vi "Is Over-Range.vi"(8 "error in (no error)":errorcluster, 10 "measurement value":dbl format="%^.2e", 11 "CS++DMM in":refnum<class "CS++DMM.lvclass">) -> (0 "error out":errorcluster, 2 "is over-range":bool, 3 "CS++DMM out":refnum<class "CS++DMM.lvclass">)   [LabVIEW 2015, in "CS++DMM.lvlib" / "CS++DMM.lvclass"]
doc: "This VI takes a measurement value that you obtain from either the Read or Fetch VIs and determines if the value is a valid measurement value or a value indicating that an over-range condition occurred. \n\nNotes:\n\n(1) If an over-range condition occurs, the measurement value contains an IEEE defined NaN (Not a Number) value indicating that an over-range condition occurred.\n\n(2) This VI does not check the instrument status."
uses:
  CS++DMM.lvclass
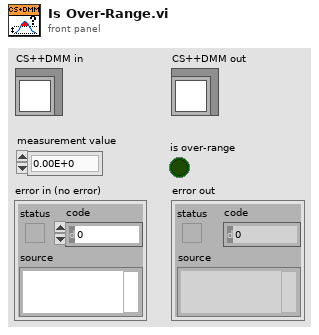
[diagram p1: front panel]
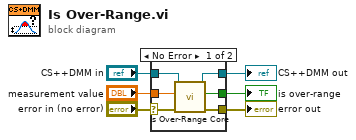
[diagram p0: block diagram]
diagram:
  n1 = case shown="No Error" "error in (no error)" {
    selector: "error in (no error)" -> [w8 w14]
    tunnel: [w7 w14] -> w5
    tunnel: [w11 w13] -> w3
    tunnel: "CS++DMM in" -> [w12 w13]
    tunnel: "measurement value" -> [w10 _]
    tunnel: [w9 _] -> w1
    frame No Error {
      n2 = call-dynamic "Is Over-Range Core.vi"("error in (no error)"=w8, "measurement value"=w10, "CS++DMM in"=w12) -> ("error out"=w7:errorcluster, "is over-range"=w9:bool, "CS++DMM out"=w11:refnum<class "CS++DMM.lvclass">)  [unwired: 6 in]
    }
    frame Error {
    }
  }
  "error out" <- w5
  "CS++DMM out" <- w3
  "is over-range" <- w1
